vi "실습 3-3 Ramp전압.vi"() -> ()   [LabVIEW 2014]
panel:
  out "웨이브폼 차트":dbl(graph)
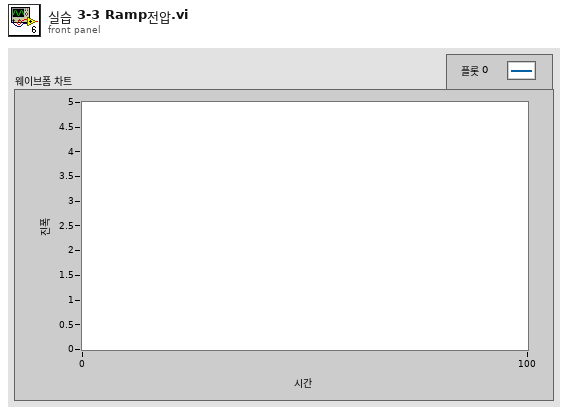
[diagram p1: front panel]
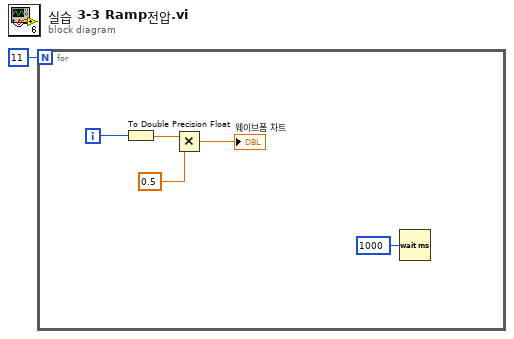
[diagram p0: block diagram]
diagram:
  n1 = for {
    N: 11 -> [_]
    i -> [w2]
    n2 = To Double Precision Float(number=w2) -> (double precision float=w6:dbl)
    n3 = Multiply(x=w6, y=0.5) -> (x*y=→"웨이브폼 차트":dbl)
    n4 = Wait (ms)(milliseconds to wait=u32 1000 ("대기 시간(ms)")) -> ()  [unwired: 1 out]
  }
